vi "ResearchStandingFrame-V1.0.vi"() -> ()   [LabVIEW 2012]
doc: "Use this template to build a simple state machine design pattern. Each state executes code and determines which state to transition to."
uses:
  controls/State.ctl
panel:
  in  "Tab Control":T1(tab)
  out "Center Mass Left Force Plate":cluster{dbl[], dbl[]}(graph)={[-7.494780644696312], [-1.1979086821741642]}
  in  "Begin":bool
  in  "stop":bool
  out "Newton Force Readings File Path":path
  in  "Newtons":bool
  out "Voltage Readings File Path":path
  out "R-FP-Z":dbl
  out "R-FP-Y":dbl
  out "R-FP-X":dbl
  out "R-LC-Z":dbl
  out "R-LC-Y":dbl
  out "R-LC-X":dbl
  out "L-LC-Z":dbl
  out "L-LC-Y":dbl
  out "L-LC-X":dbl
  out "L-FP-X":dbl
  out "L-FP-Y":dbl
  out "L-FP-Z":dbl
  out "String":string caption="Display Unit"
  out "Left Force Plate Z":dbl(slide)=0.4283867154785348 scale=0.0..300.0
  out "Right Force Plate Z":dbl(slide)=1.117665643201773 scale=0.0..300.0
  out "Center Mass Right Force Plate":cluster{dbl[], dbl[]}(graph)
  out "Right Load Cell":cluster{dbl[], dbl[]}(graph)={[0.0, -0.0006862149399022939, 0.0, 0.0], [0.0, 0.005798023167495851, 0.0, 0.0]}
  out "Right Load Cell Z":dbl(slide)=0.024398753418748073 scale=-50.0..300.0
  out "Left Load Cell Z":dbl(slide)=-0.05310519238420746 scale=-50.0..300.0
  out "Left Load Cell":cluster{dbl[], dbl[]}(graph)={[0.0, -0.0004854170425343219, 0.0, 0.0], [0.0, -0.002818533162237429, 0.0, 0.0]}
  out "Amplitude Unit":string
  out "Right Force PLate Z":dbl(graph)
  out "Left Force Plate Z":dbl(graph)
  out "Right Load Cell Z":dbl(graph)
  out "Right Load Cell Y":dbl(graph)
  out "Right Load Cell X":dbl(graph)
  out "Left Load Cell Z":dbl(graph)
  out "Left Load Cell Y":dbl(graph)
  out "Left Load Cell X":dbl(graph)
  out "Amplitude Unit":string
  out "Baseline Out":dbl[](array[numeric])
  out "Voltages":dbl[](array[numeric])
  in  "Baseline":bool
  # "Left Load Cell X\n\nLeft Load Cell Y\n\n\nLeft Load Cell Z\n\nRight Load Cell X\n\n\nRight Load Cell Y\n\nRight Load Cell Z\n\n\nLeft Force Plate X1\n\nLeft Force Plate X2\n\n\nLeft Force Plate Y1\n\nLeft Force PLate Y2\n\n\nLeft Force Plate Z1\n\nLeft Force Plate Z2\n\n\nLeft Force Plate Z3\n\nLeft Force Plate Z4\n\n\nRight Force Plate X1\n\nRight Force Plate X2\n\n\nRight Force Plate Y1\n\nRight Force PLate Y2\n\n\nRight Force Plate Z1\n\nRight Force Plate Z2\n\n\nRight Force Plate Z3\n\nRight Force Plate Z4"
  # "DAQ Board Connections"
  # "LX\nLY\nLZ\nRX\nRY\nRZ\nLFX12\nLFX34\nLFY14\nLFY23\nLFZ1\nLFZ2\nLFZ3\nLFZ4\nRFX12\nRFX34\nRFY14\nRFY23\nRFZ1\nRFZ2\nRFZ3\nRFZ4"
  # "32\n33\n34\n35\n36\n37\n0\n1\n2\n3\n4\n5\n6\n7\n16\n17\n18\n19\n20\n21\n22\n23"
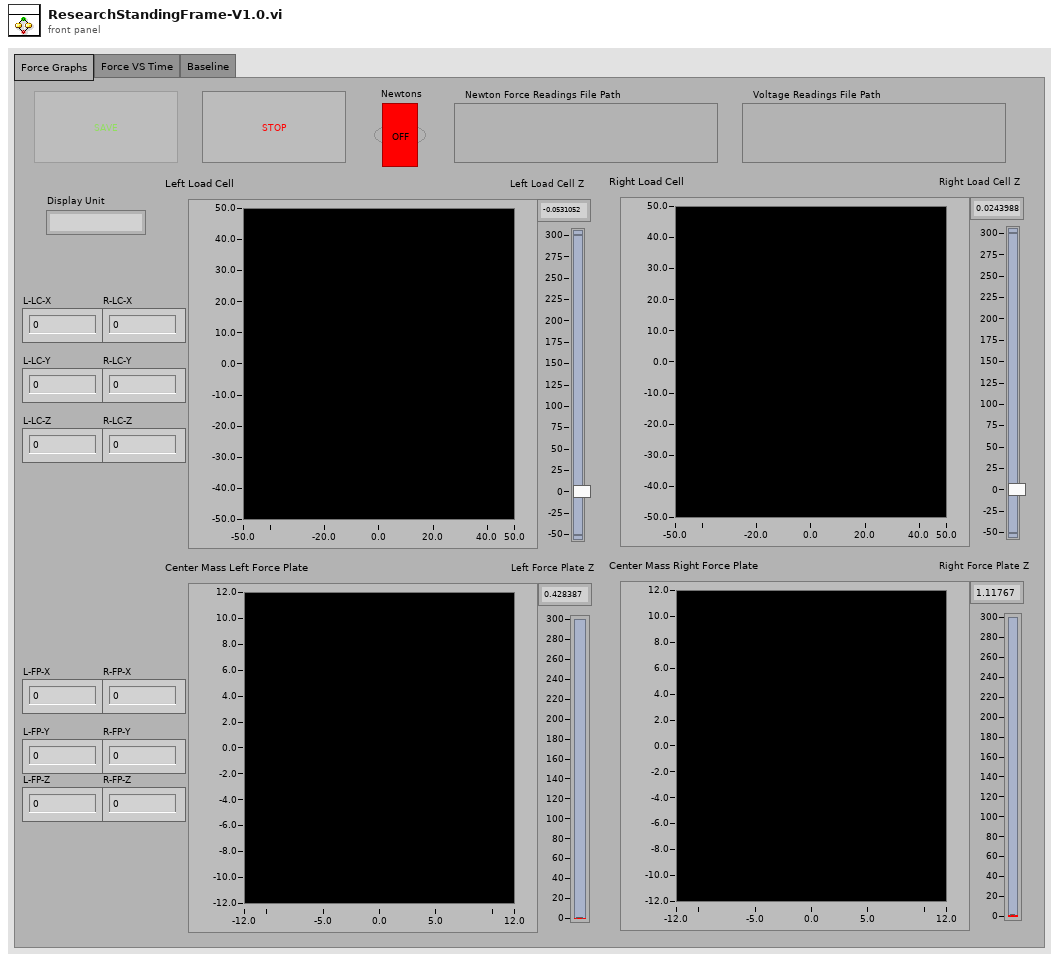
[diagram p1: front panel]
types:
  T1 = enum32{"Force Graphs", "Force VS Time", "Baseline"}
  T2 = typedef "State.ctl" = enum16{"Initialize", "Idle", "Save", "Main", "Stop"}
  T3 = enum16{"open", "replace", "create", "open or create", "replace or create", "replace or create with confirmation"}
  T4 = enum8{"Enabled", "Disabled", "Disabled and Grayed Out"}
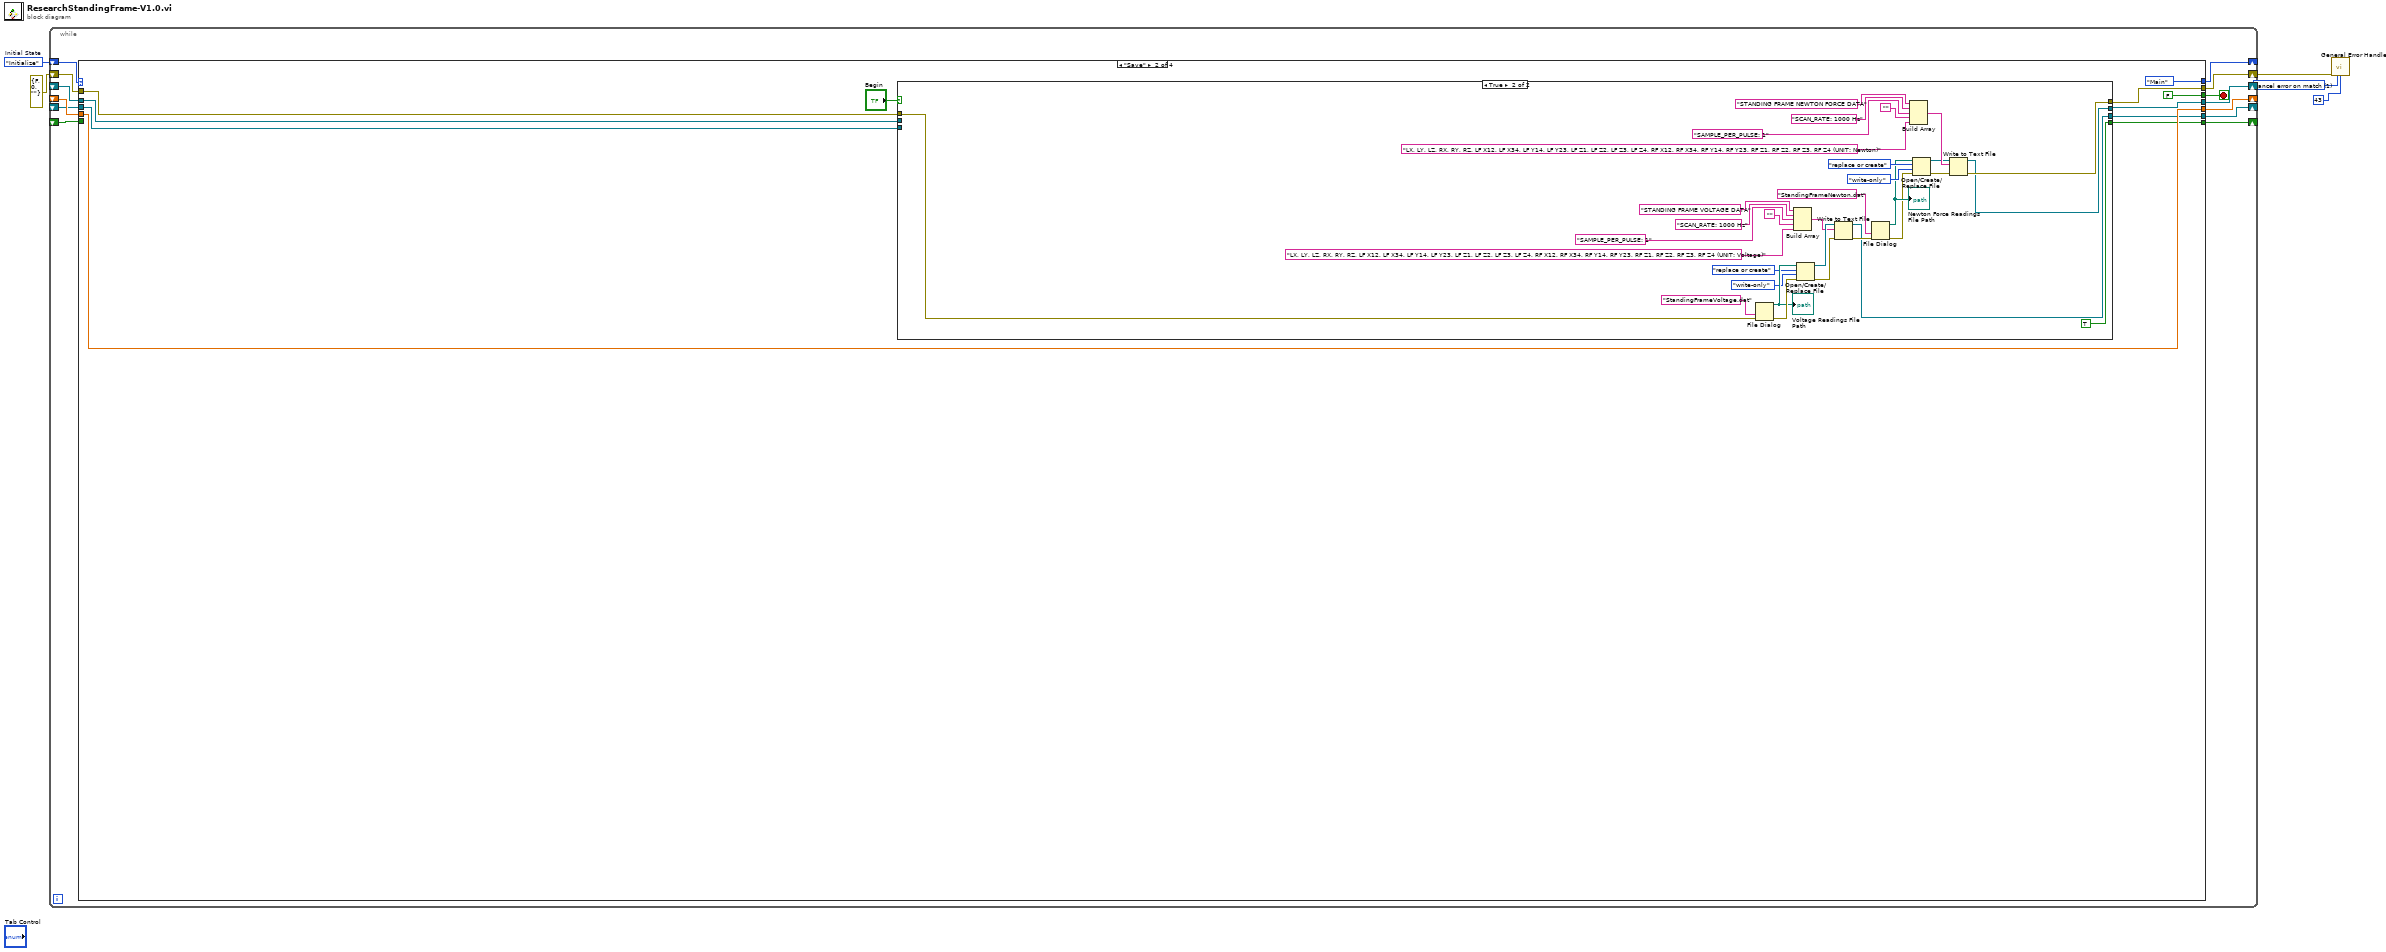
[diagram p0: block diagram]
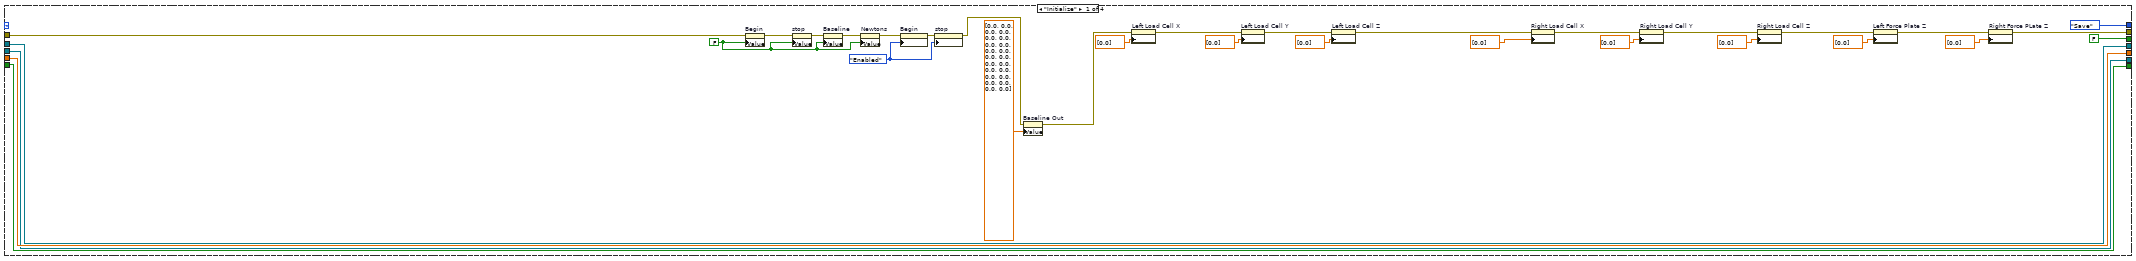
[diagram p2: hidden frame]
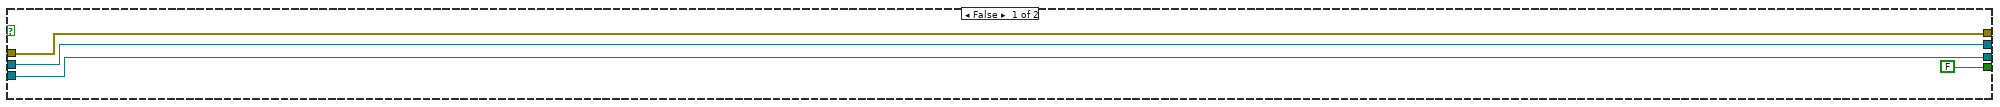
[diagram p3: hidden frame]
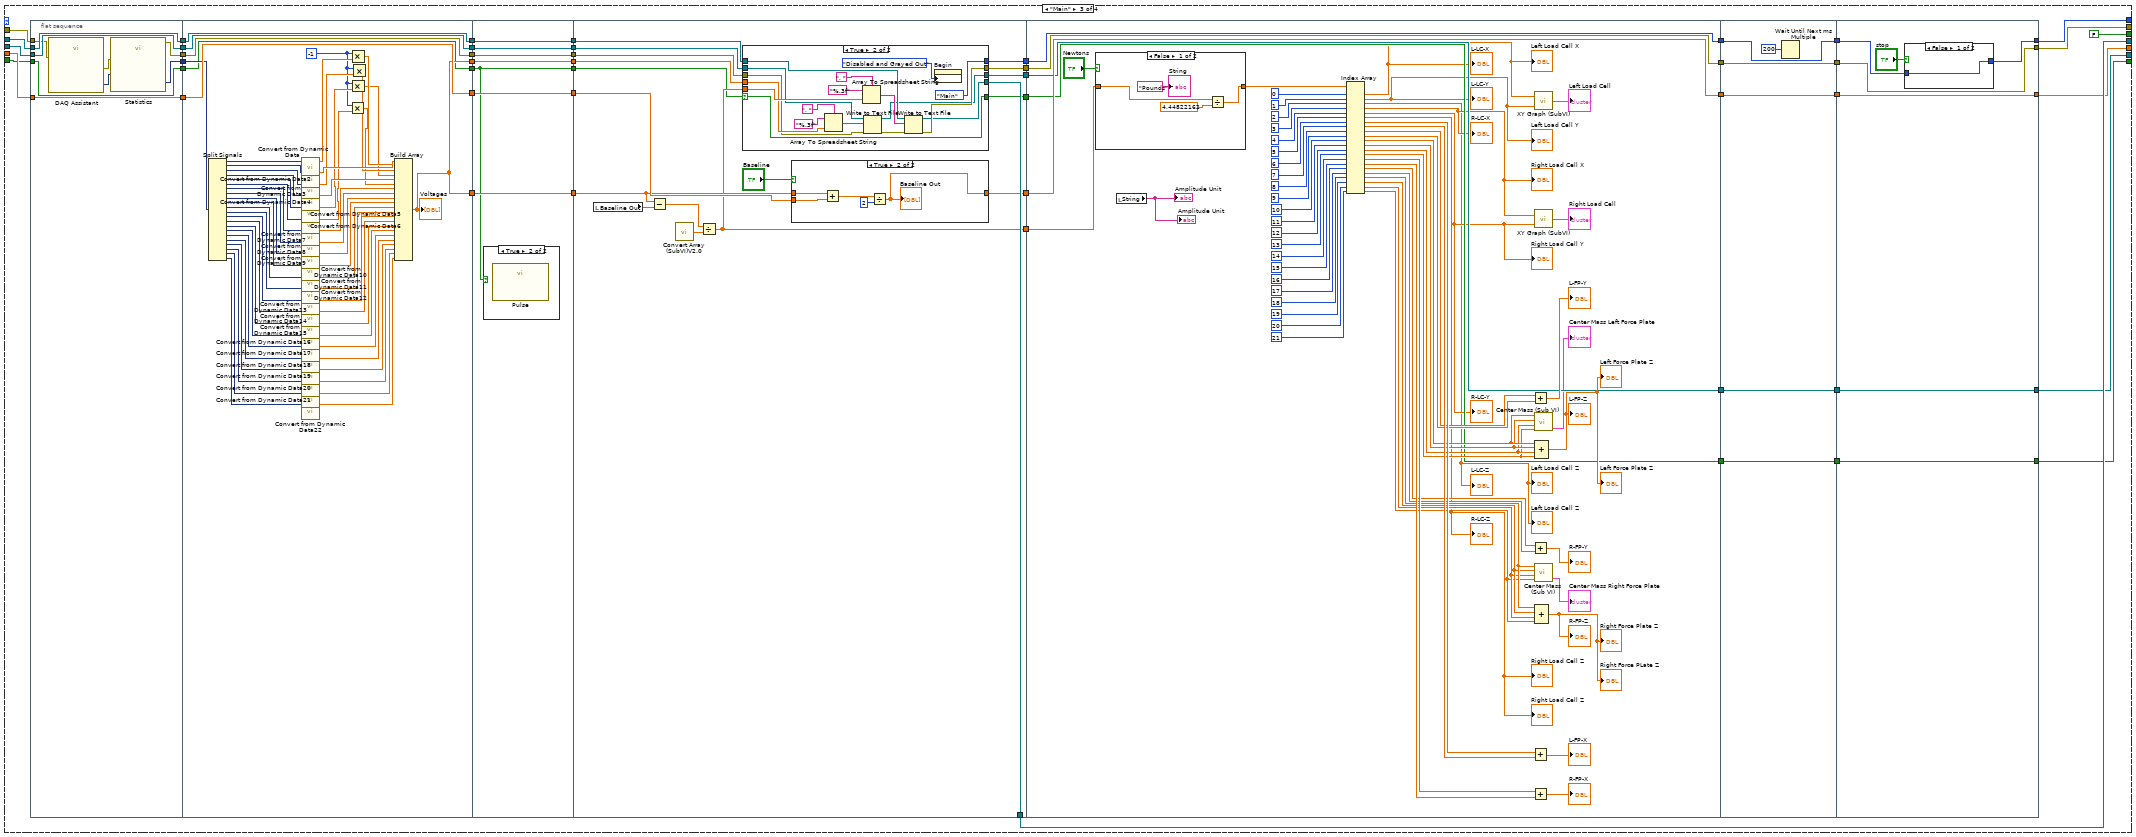
[diagram p4: hidden frame]
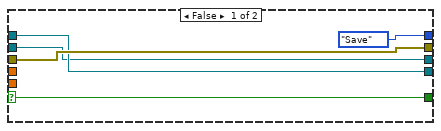
[diagram p6: hidden frame]
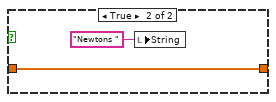
[diagram p8: hidden frame]
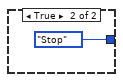
[diagram p9: hidden frame]
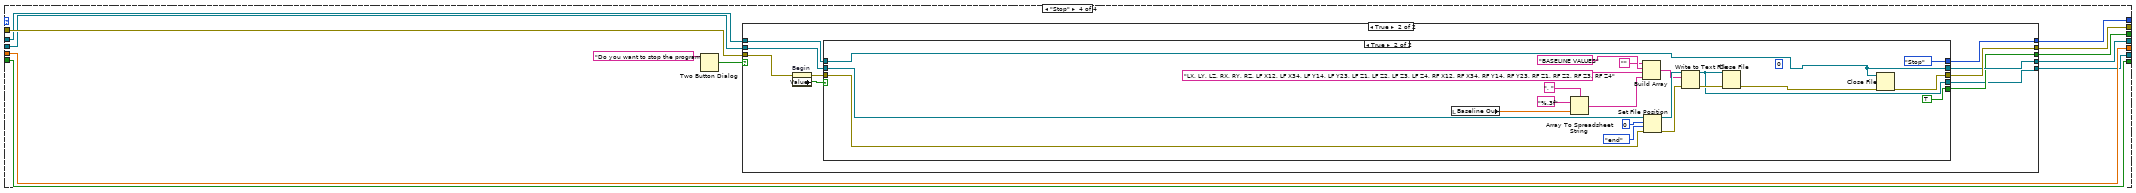
[diagram p10: hidden frame]
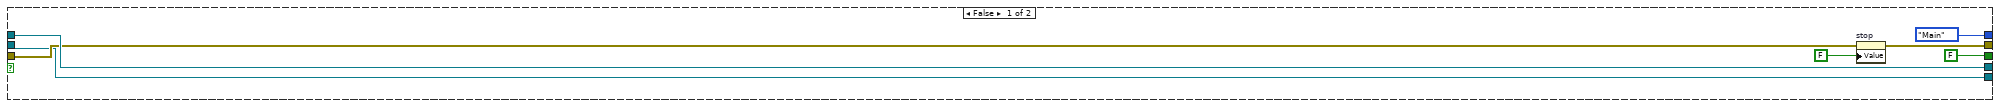
[diagram p11: hidden frame]
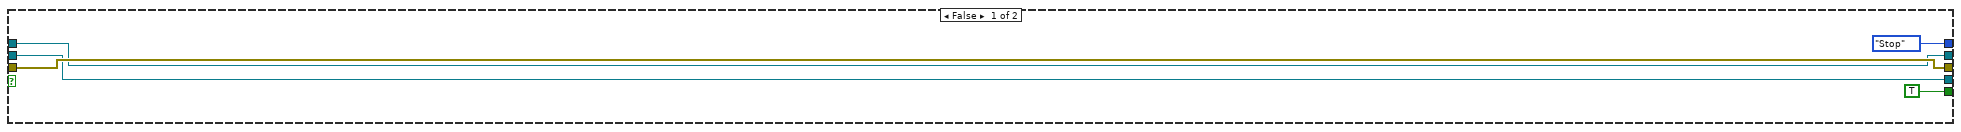
[diagram p12: hidden frame]
diagram:
  w1 = 1 items=["no exception", "cancel error on match", "set error on match"] ("[exception action] (none:0)")
  w5 = State."Initialize"  # Initial State
  n1 = while {
    shift-right: [w17] -> _
    shift-left: w5 -> [w18]
    shift-right: [w12] -> w3
    shift-left: errorcluster {"status"=FALSE, "code"=0, "source"=""} ("error out") -> [w16]
    shift-right: [w14] -> _
    shift-left: _ -> [w13]
    shift-right: [w10] -> _
    shift-left: _ -> [w11]
    shift-right: [w9] -> _
    shift-left: _ -> [w8]
    shift-right: [w7] -> _
    shift-left: _ -> [w6]
    stop <- w15 stop-if-true
    n2 = case shown="\"Save\"" w18 {
      tunnel: [State."Save" ("Next State") State."Main" ("Next State") w144 w359] -> w17
      tunnel: [FALSE ("T button?") FALSE FALSE ("T button?") w358] -> w15
      tunnel: w16 -> [w45 w60 w146 w357]
      tunnel: [w49 w59 w139 w354] -> w14
      tunnel: w13 -> [w49 w56 w145 w355]
      tunnel: [w21 w58 w131 w356] -> w12
      tunnel: w11 -> [w44 w55 w129 w353]
      tunnel: [w44 w55 w125 w353] -> w10
      tunnel: [w41 w52 w124 w352] -> w9
      tunnel: w8 -> [w41 w54 w119 w351]
      tunnel: [w19 w53 w116 w350] -> w7
      tunnel: w6 -> [w19 _ w117 w350]
      frame "Initialize" {
        w38 = FALSE ("Begin")
        w48 = T4."Enabled" ("Disabled")
        n3 = property on="Begin" class="Bool (strict)"(error in=w45, "Value"=w38) -> (error out=w47:errorcluster)  [unwired: 1 in, 1 out]
        n4 = property on="stop" class="Bool (strict)"(error in=w47, "Value"=w38) -> (error out=w43:errorcluster)  [unwired: 1 in, 1 out]
        n5 = property on="Baseline" class="Bool (strict)"(error in=w43, "Value"=w38) -> (error out=w40:errorcluster)  [unwired: 1 in, 1 out]
        n6 = property on="Newtons" class="Bool (strict)"(error in=w40, "Value"=w38) -> (error out=w39:errorcluster)  [unwired: 1 in, 1 out]
        n7 = property on="Begin" class="Bool (strict)"(error in=w39, "DisabledEnum"=w48) -> (error out=w46:errorcluster)  [unwired: 1 in, 1 out]
        n8 = property on="stop" class="Bool (strict)"(error in=w46, "DisabledEnum"=w48) -> (error out=w20:errorcluster)  [unwired: 1 in, 1 out]
        n9 = property on="Baseline Out" class="Arr (strict)"(error in=w20, "Value"=dbl[] [0.0, 0.0, 0.0, 0.0, 0.0, 0.0, 0.0, 0.0, 0.0, 0.0, 0.0, 0.0, 0.0, 0.0, 0.0, 0.0, 0.0, 0.0, 0.0, 0.0, 0.0, 0.0] ("Baseline Out")) -> (error out=w29:errorcluster)  [unwired: 1 in, 1 out]
        n10 = property on="Left Load Cell X" class="WFChart (strict)"(error in=w29, "History Data"=dbl[] [0.0]) -> (error out=w28:errorcluster)  [unwired: 1 in, 1 out]
        n11 = property on="Left Load Cell Y" class="WFChart (strict)"(error in=w28, "History Data"=dbl[] [0.0]) -> (error out=w27:errorcluster)  [unwired: 1 in, 1 out]
        n12 = property on="Left Load Cell Z" class="WFChart (strict)"(error in=w27, "History Data"=dbl[] [0.0]) -> (error out=w26:errorcluster)  [unwired: 1 in, 1 out]
        n13 = property on="Right Load Cell X" class="WFChart (strict)"(error in=w26, "History Data"=dbl[] [0.0]) -> (error out=w25:errorcluster)  [unwired: 1 in, 1 out]
        n14 = property on="Right Load Cell Y" class="WFChart (strict)"(error in=w25, "History Data"=dbl[] [0.0]) -> (error out=w24:errorcluster)  [unwired: 1 in, 1 out]
        n15 = property on="Right Load Cell Z" class="WFChart (strict)"(error in=w24, "History Data"=dbl[] [0.0]) -> (error out=w23:errorcluster)  [unwired: 1 in, 1 out]
        n16 = property on="Left Force Plate Z" class="WFChart (strict)"(error in=w23, "History Data"=dbl[] [0.0]) -> (error out=w22:errorcluster)  [unwired: 1 in, 1 out]
        n17 = property on="Right Force PLate Z" class="WFChart (strict)"(error in=w22, "History Data"=dbl[] [0.0]) -> (error out=w21:errorcluster)  [unwired: 1 in, 1 out]
      }
      frame "Save" {
        n18 = case shown="True" "Begin" {
          tunnel: w60 -> [w66 w78]
          tunnel: [w65 w92] -> w59
          tunnel: [w66 w94] -> w58
          tunnel: w56 -> [w65 _]
          tunnel: [w64 w76] -> w52
          tunnel: w54 -> [w64 _]
          tunnel: [FALSE TRUE] -> w53
          frame False {
          }
          frame True {
            n19 = File Dialog(8:w78, 9:"StandingFrameVoltage.dat" ("default name")) -> (0:w86:errorcluster, 3:w84:path)  [unwired: 1 in, 6 out]
            "Voltage Readings File Path" <- w84
            n20 = Build Array("STANDING FRAME VOLTAGE DATA", "SCAN_RATE: 1000 Hz", "SAMPLE_PER_PULSE: 1", "", "LX, LY, LZ, RX, RY, RZ, LF X12, LF X34, LF Y14, LF Y23, LF Z1, LF Z2, LF Z3, LF Z4, RF X12, RF X34, RF Y14, RF Y23, RF Z1, RF Z2, RF Z3, RF Z4 (UNIT: Voltage)") -> (w82:string[])
            n21 = Open/Create/Replace File(file path (use dialog)=w84, error in=w86, operation (0:open)=T3."replace or create", access (0:read/write)=enum16{"read/write", "read-only", "write-only"}."write-only") -> (refnum out=w83:refnum<file>, error out=w87:errorcluster)  [unwired: 3 out]
            n22 = Write to Text File(file (use dialog)=w83, text=w82, error in=w87) -> (refnum out=w76:refnum<file>, error out=w77:errorcluster)  [unwired: 1 in, 1 out]
            n23 = File Dialog(8:w77, 9:"StandingFrameNewton.dat" ("default name")) -> (0:w89:errorcluster, 3:w91:path)  [unwired: 1 in, 6 out]
            "Newton Force Readings File Path" <- w91
            n24 = Build Array("STANDING FRAME NEWTON FORCE DATA", "SCAN_RATE: 1000 Hz", "SAMPLE_PER_PULSE: 1", "", "LX, LY, LZ, RX, RY, RZ, LF X12, LF X34, LF Y14, LF Y23, LF Z1, LF Z2, LF Z3, LF Z4, RF X12, RF X34, RF Y14, RF Y23, RF Z1, RF Z2, RF Z3, RF Z4 (UNIT: Newton)") -> (w95:string[])
            n25 = Open/Create/Replace File(file path (use dialog)=w91, error in=w89, operation (0:open)=T3."replace or create", access (0:read/write)=enum16{"read/write", "read-only", "write-only"}."write-only") -> (refnum out=w93:refnum<file>, error out=w88:errorcluster)  [unwired: 3 out]
            n26 = Write to Text File(file (use dialog)=w93, text=w95, error in=w88) -> (refnum out=w92:refnum<file>, error out=w94:errorcluster)  [unwired: 1 in, 1 out]
          }
        }
      }
      frame "Main" {
        n27 = flat-sequence {
          tunnel: w146 -> [w150]
          tunnel: w145 -> [w153]
          tunnel: [w155] -> w142
          tunnel: [w154] -> w141
          tunnel: [w153] -> w140
          tunnel: [w152] -> w130
          tunnel: w129 -> [w152]
          tunnel: [w151] -> w120
          tunnel: w119 -> [w151]
          tunnel: [w149] -> w118
          tunnel: w117 -> [w149]
          tunnel: w142 -> [w187]
          tunnel: [w187] -> w110
          tunnel: w141 -> [w210]
          tunnel: w140 -> [w186]
          tunnel: [w186] -> w112
          tunnel: [w211] -> w108
          tunnel: w130 -> [w211]
          tunnel: [w173] -> w106
          tunnel: [w173] -> w104
          tunnel: [w172] -> w102
          tunnel: w120 -> [w172]
          tunnel: [w167] -> w100
          tunnel: w118 -> [w167]
          tunnel: w112 -> [w218]
          tunnel: [w218] -> w111
          tunnel: w110 -> [w217]
          tunnel: [w217] -> w109
          tunnel: w108 -> [w216]
          tunnel: [w216] -> w107
          tunnel: w106 -> [w215]
          tunnel: [w215] -> w105
          tunnel: w104 -> [w214]
          tunnel: [w214] -> w103
          tunnel: w102 -> [w213]
          tunnel: [w213] -> w101
          tunnel: w100 -> [w212]
          tunnel: [w212] -> w99
          tunnel: [w232] -> w138
          tunnel: [w235] -> w139
          tunnel: w111 -> [w233]
          tunnel: w109 -> [w234]
          tunnel: [w231] -> w137
          tunnel: [w221] -> w136
          tunnel: w107 -> [w230]
          tunnel: w105 -> [w228]
          tunnel: [w227] -> w128
          tunnel: w103 -> [w226]
          tunnel: [w225] -> w121
          tunnel: w101 -> [w224]
          tunnel: w99 -> [w220]
          tunnel: [w219] -> w113
          tunnel: w138 -> [w328]
          tunnel: [w328] -> w135
          tunnel: w137 -> [w275]
          tunnel: w136 -> [w326]
          tunnel: [w275] -> w133
          tunnel: w128 -> [w292]
          tunnel: [w292] -> w127
          tunnel: [w291] -> w122
          tunnel: w121 -> [w291]
          tunnel: [w276] -> w114
          tunnel: w113 -> [w276]
          tunnel: w135 -> [w340]
          tunnel: [w340] -> w134
          tunnel: w133 -> [w338]
          tunnel: [w338] -> w132
          tunnel: w127 -> [w337]
          tunnel: [w337] -> w126
          tunnel: [w336] -> w123
          tunnel: w122 -> [w336]
          tunnel: [w335] -> w115
          tunnel: w114 -> [w335]
          tunnel: [w347] -> w144
          tunnel: w134 -> [w345]
          tunnel: w132 -> [w344]
          tunnel: [w344] -> w131
          tunnel: w126 -> [w343]
          tunnel: [w343] -> w125
          tunnel: [w342] -> w124
          tunnel: w123 -> [w342]
          tunnel: [w341] -> w116
          tunnel: w115 -> [w341]
          frame #0 {
            n28 = call "DAQ Assistant"("error in"=w150) -> ("data"=w147:dynamicdata, "error out"=w148:errorcluster)  [unwired: 16 in, 1 out]
            n29 = call "Statistics"("Signals"=w147, "error in (no error)"=w148) -> ("Arithmetic Mean"=w154:dynamicdata, "error out"=w155:errorcluster)  [unwired: 24 in]
          }
          frame #1 {
            w158 = -1
            n30 = Split Signals(w210) -> (w209:dynamicdata, w208:dynamicdata, w207:dynamicdata, w206:dynamicdata, w205:dynamicdata, w204:dynamicdata, w203:dynamicdata, w202:dynamicdata, w201:dynamicdata, w200:dynamicdata, w199:dynamicdata, w198:dynamicdata, w197:dynamicdata, w196:dynamicdata, w195:dynamicdata, w194:dynamicdata, w193:dynamicdata, w192:dynamicdata, w191:dynamicdata, w190:dynamicdata, w189:dynamicdata, w188:dynamicdata)  [unwired: 22 in]
            n31 = call "Convert from Dynamic Data"("Dynamic Data Type"=w209) -> ("Scalar"=w165:dbl)  [unwired: 3 in]
            n32 = call "Convert from Dynamic Data2"("Dynamic Data Type"=w208) -> ("Scalar"=w166:dbl)  [unwired: 3 in]
            n33 = call "Convert from Dynamic Data3"("Dynamic Data Type"=w207) -> ("Scalar"=w163:dbl)  [unwired: 3 in]
            n34 = call "Convert from Dynamic Data4"("Dynamic Data Type"=w206) -> ("Scalar"=w161:dbl)  [unwired: 3 in]
            n35 = call "Convert from Dynamic Data5"("Dynamic Data Type"=w205) -> ("Scalar"=w160:dbl)  [unwired: 3 in]
            n36 = call "Convert from Dynamic Data6"("Dynamic Data Type"=w204) -> ("Scalar"=w157:dbl)  [unwired: 3 in]
            n37 = call "Convert from Dynamic Data7"("Dynamic Data Type"=w203) -> ("Scalar"=w174:dbl)  [unwired: 3 in]
            n38 = call "Convert from Dynamic Data8"("Dynamic Data Type"=w202) -> ("Scalar"=w175:dbl)  [unwired: 3 in]
            n39 = call "Convert from Dynamic Data9"("Dynamic Data Type"=w201) -> ("Scalar"=w176:dbl)  [unwired: 3 in]
            n40 = call "Convert from Dynamic Data10"("Dynamic Data Type"=w200) -> ("Scalar"=w177:dbl)  [unwired: 3 in]
            n41 = call "Convert from Dynamic Data11"("Dynamic Data Type"=w199) -> ("Scalar"=w171:dbl)  [unwired: 3 in]
            n42 = call "Convert from Dynamic Data12"("Dynamic Data Type"=w198) -> ("Scalar"=w170:dbl)  [unwired: 3 in]
            n43 = call "Convert from Dynamic Data13"("Dynamic Data Type"=w197) -> ("Scalar"=w178:dbl)  [unwired: 3 in]
            n44 = call "Convert from Dynamic Data14"("Dynamic Data Type"=w196) -> ("Scalar"=w169:dbl)  [unwired: 3 in]
            n45 = call "Convert from Dynamic Data15"("Dynamic Data Type"=w195) -> ("Scalar"=w168:dbl)  [unwired: 3 in]
            n46 = call "Convert from Dynamic Data16"("Dynamic Data Type"=w194) -> ("Scalar"=w179:dbl)  [unwired: 3 in]
            n47 = call "Convert from Dynamic Data17"("Dynamic Data Type"=w193) -> ("Scalar"=w180:dbl)  [unwired: 3 in]
            n48 = call "Convert from Dynamic Data18"("Dynamic Data Type"=w192) -> ("Scalar"=w181:dbl)  [unwired: 3 in]
            n49 = call "Convert from Dynamic Data19"("Dynamic Data Type"=w191) -> ("Scalar"=w182:dbl)  [unwired: 3 in]
            n50 = call "Convert from Dynamic Data20"("Dynamic Data Type"=w190) -> ("Scalar"=w183:dbl)  [unwired: 3 in]
            n51 = call "Convert from Dynamic Data21"("Dynamic Data Type"=w189) -> ("Scalar"=w184:dbl)  [unwired: 3 in]
            n52 = call "Convert from Dynamic Data22"("Dynamic Data Type"=w188) -> ("Scalar"=w185:dbl)  [unwired: 3 in]
            n53 = Multiply(x=w158, y=w157) -> (x*y=w156:dbl)
            n54 = Multiply(x=w158, y=w165) -> (x*y=w164:dbl)
            n55 = Multiply(x=w158, y=w160) -> (x*y=w159:dbl)
            n56 = Multiply(x=w158, y=w163) -> (x*y=w162:dbl)
            n57 = Build Array(w166, w164, w162, w159, w161, w156, w174, w175, w176, w177, w171, w170, w178, w169, w168, w179, w180, w181, w182, w183, w184, w185) -> (w173:dbl[])
            "Voltages" <- w173
          }
          frame #2 {
            n58 = case shown="True" w212 {
              frame False {
              }
              frame True {
                n59 = call "Pulse"() -> ()  [unwired: 18 in, 2 out]
              }
            }
          }
          frame #3 {
            n60 = local read "Baseline Out"() -> (w229:dbl[])
            n61 = Subtract(x=w228, y=w229) -> (x-y=w223:dbl[])
            n62 = call "Convert Array  (SubVI)V2.0.vi"() -> ("Conversion Array"=w222:dbl[])  [unwired: 1 in]
            n63 = Divide(x=w223, y=w222) -> (x/y=w221:dbl[])
            n64 = case shown="True" w220 {
              selector: w220 -> [w237 w242]
              tunnel: [w241 w256] -> w231
              tunnel: [w239 w255] -> w235
              tunnel: w234 -> [w241 w246]
              tunnel: [State."Save" ("(Value Not Used)") State."Main" ("(Value Not Used)")] -> w232
              tunnel: w233 -> [w239 w252]
              tunnel: w221 -> [_ w253]
              tunnel: w226 -> [_ w247]
              tunnel: [w238 w244] -> w225
              tunnel: w224 -> [w238 w243]
              tunnel: [w237 w242] -> w219
              frame False {
              }
              frame True {
                n65 = Array To Spreadsheet String(delimiter (Tab)=", ", array=w247, 3:"%.3f") -> (spreadsheet string=w248:string)
                n66 = Array To Spreadsheet String(delimiter (Tab)=", ", array=w253, 3:"%.3f") -> (spreadsheet string=w259:string)
                n67 = Write to Text File(file (use dialog)=w243, text=w248, error in=w246) -> (refnum out=w244:refnum<file>, error out=w245:errorcluster)  [unwired: 1 in, 1 out]
                n68 = Write to Text File(file (use dialog)=w252, text=w259, error in=w245) -> (refnum out=w255:refnum<file>, error out=w256:errorcluster)  [unwired: 1 in, 1 out]
                n69 = property on="Begin" class="Bool (strict)"("DisabledEnum"=T4."Disabled and Grayed Out" ("Disabled")) -> ()  [unwired: 2 in, 2 out]
              }
            }
            n70 = case shown="True" "Baseline" {
              tunnel: w230 -> [_ w261]
              tunnel: w228 -> [w260 w263]
              tunnel: [w260 w262] -> w227
              frame False {
              }
              frame True {
                n71 = Add(x=w263, y=w261) -> (x+y=w265:dbl[])
                n72 = Divide(x=w265, y=2) -> (x/y=w262:dbl[])
                "Baseline Out" <- w262
              }
            }
          }
          frame #4 {
            n73 = case shown="False" "Newtons" {
              tunnel: w326 -> [w331 w333]
              tunnel: [w330 w333] -> w325
              frame False {
                n74 = Divide(x=w331, y=4.44822162) -> (x/y=w330:dbl[])
                "String" <- "Pounds" ("String")
              }
              frame True {
                n75 = local write "String"("Newtons " ("String")) -> ()
              }
            }
            n76 = local read "String"() -> (→"Amplitude Unit" →"Amplitude Unit":string)
            n77 = Index Array(array=w325, index #1=0 ("index (row)"), index #2=1 ("index (row)"), index #3=2 ("index (row)"), index #4=3 ("index (row)"), index #5=4 ("index (row)"), index #6=5 ("index (row)"), index #7=6 ("index (row)"), index #8=7 ("index (row)"), index #9=8 ("index (row)"), index #10=9 ("index (row)"), index #11=10 ("index (row)"), index #12=11 ("index (row)"), index #13=12 ("index (row)"), index #14=13 ("index (row)"), index #15=14 ("index (row)"), index #16=15 ("index (row)"), index #17=16 ("index (row)"), index #18=17 ("index (row)"), index #19=18 ("index (row)"), index #20=19 ("index (row)"), index #21=20 ("index (row)"), index #22=21 ("index (row)")) -> (element #1=w269:dbl, element #2=w270:dbl, element #3=→"L-LC-Z" →"Left Load Cell Z" →"Left Load Cell Z":dbl, element #4=w271:dbl, element #5=w272:dbl, element #6=→"R-LC-Z" →"Right Load Cell Z" →"Right Load Cell Z":dbl, element #7=w302:dbl, element #8=w301:dbl, element #9=w299:dbl, element #10=w298:dbl, element #11=w286:dbl, element #12=w285:dbl, element #13=w284:dbl, element #14=w283:dbl, element #15=w296:dbl, element #16=w295:dbl, element #17=w294:dbl, element #18=w293:dbl, element #19=w282:dbl, element #20=w281:dbl, element #21=w280:dbl, element #22=w279:dbl)
            "L-LC-X" <- w269
            "L-LC-Y" <- w270
            "R-LC-X" <- w271
            "R-LC-Y" <- w272
            "Left Load Cell X" <- w269
            "Left Load Cell Y" <- w270
            "Right Load Cell X" <- w271
            "Right Load Cell Y" <- w272
            n78 = Add(x=w299, y=w298) -> (x+y=→"L-FP-Y":dbl)
            n79 = Add(x=w294, y=w293) -> (x+y=→"R-FP-Y":dbl)
            n80 = Add(x=w302, y=w301) -> (x+y=→"L-FP-X":dbl)
            n81 = Add(x=w296, y=w295) -> (x+y=→"R-FP-X":dbl)
            n82 = call "Center Mass (Sub VI).vi"("Z4"=w283, "Z3"=w284, "Z2"=w285, "Z1"=w286) -> ("XY Graph"=→"Center Mass Left Force Plate":cluster{dbl[], dbl[]})  [unwired: 2 in]
            n83 = call "Center Mass (Sub VI).vi"("Z4"=w279, "Z3"=w280, "Z2"=w281, "Z1"=w282) -> ("XY Graph"=→"Center Mass Right Force Plate":cluster{dbl[], dbl[]})  [unwired: 2 in]
            n84 = call "XY Graph (SubVI).vi"("Y"=w270, "X"=w269) -> ("XY Graph"=→"Left Load Cell":cluster{"array":dbl[], "array":dbl[]})
            n85 = call "XY Graph (SubVI).vi"("Y"=w272, "X"=w271) -> ("XY Graph"=→"Right Load Cell":cluster{"array":dbl[], "array":dbl[]})
            n86 = Compound Arithmetic op=ADD(w286, w285, w284, w283) -> (→"L-FP-Z" →"Left Force Plate Z" →"Left Force Plate Z":dbl)
            n87 = Compound Arithmetic op=ADD(w282, w281, w280, w279) -> (→"R-FP-Z" →"Right Force PLate Z" →"Right Force Plate Z":dbl)
          }
          frame #5 {
            n88 = Wait Until Next ms Multiple(millisecond multiple=u32 200) -> ()  [unwired: 1 out]
          }
          frame #6 {
            n89 = case shown="False" "stop" {
              tunnel: [w348 State."Stop" ("(Value Not Used)")] -> w347
              tunnel: w345 -> [w348 _]
              frame False {
              }
              frame True {
              }
            }
          }
        }
      }
      frame "Stop" {
        n90 = Two Button Dialog(message="Do you want to stop the program?") -> (T button?=w360:bool)  [unwired: 2 in]
        n91 = case shown="True" w360 {
          tunnel: [FALSE w374] -> w358
          tunnel: [State."Main" ("(Value Not Used)") w375] -> w359
          tunnel: w357 -> [w363 w373]
          tunnel: [w364 w378] -> w356
          tunnel: w355 -> [w366 w377]
          tunnel: [w366 w376] -> w354
          tunnel: [w362 w370] -> w352
          tunnel: w351 -> [w362 w369]
          frame False {
            n92 = property on="stop" class="Bool (strict)"(error in=w363, "Value"=FALSE ("stop")) -> (error out=w364:errorcluster)  [unwired: 1 in, 1 out]
          }
          frame True {
            n93 = property on="Begin" class="Bool (strict)"(error in=w373) -> (error out=w372:errorcluster, "Value"=w371:bool)  [unwired: 1 in, 1 out]
            n94 = case shown="True" w371 {
              tunnel: w372 -> [w381 w388]
              tunnel: [w381 w397] -> w378
              tunnel: w377 -> [w380 w386]
              tunnel: [w380 w386] -> w376
              tunnel: [State."Stop" ("(Value Not Used)") State."Stop" ("(Value Not Used)")] -> w375
              tunnel: [TRUE TRUE] -> w374
              tunnel: [w379 w391] -> w370
              tunnel: w369 -> [w379 w390]
              frame False {
              }
              frame True {
                (unwired) 0 ("pos offset (0)")
                n95 = local read "Baseline Out"() -> (w400:dbl[])
                n96 = Array To Spreadsheet String(delimiter (Tab)=", ", array=w400, 3:"%.3f") -> (spreadsheet string=w384:string)
                n97 = Build Array("", "BASELINE VALUES", "LX, LY, LZ, RX, RY, RZ, LF X12, LF X34, LF Y14, LF Y23, LF Z1, LF Z2, LF Z3, LF Z4, RF X12, RF X34, RF Y14, RF Y23, RF Z1, RF Z2, RF Z3, RF Z4", w384) -> (w389:string[])
                n98 = Set File Position(offset (in bytes) (0)=0 ("pos offset (0)"), refnum=w390, from (0:start)=enum16{"start", "end", "current"}."end" ("pos mode (0:2)"), error in=w388) -> (refnum out=w394:refnum<file>, error out=w395:errorcluster)
                n99 = Write to Text File(file (use dialog)=w394, text=w389, error in=w395) -> (refnum out=w391:refnum<file>, error out=w396:errorcluster)  [unwired: 1 in, 1 out]
                n100 = Close File(refnum=w391, error in=w396) -> (error out=w387:errorcluster)  [unwired: 1 out]
                n101 = Close File(refnum=w386, error in=w387) -> (error out=w397:errorcluster)  [unwired: 1 out]
              }
            }
          }
        }
      }
    }
  }
  n102 = call <vilib>:"General Error Handler.vi"("error in (no error)"=w3, "[exception action] (none:0)"=w1, "[exception code]"=43) -> ()  [unwired: 8 in, 5 out]
